vi "draw_position_overlay.vi"(7 "pixel look-up mode":T1, 8 "error in (no error)":errorcluster, 9 "pixel positions":T2[](array[typedef]), 10 "frame index":i32, 11 "ImageCollection in":refnum<class "ImageCollection.lvclass">) -> (0 "error out":errorcluster, 2 "Image.lvclass":refnum<class "Image.lvclass">, 3 "ImageCollection out":refnum<class "ImageCollection.lvclass">)   [LabVIEW 2010, in "ImageCollection.lvclass"]
uses:
  ImageCollection.lvclass
  Image/Image/Image.lvclass
  pixel_position_cluster.ctl
  enumerations/pixel_lookup_mode_enum.ctl
  Image/Image/pixel_position_cluster.ctl
  Image/Image/pixel_positions_cluster.ctl
  ImageCollection.lvclass/ImageCollection.ctl
panel:
  out "is line on current plane?":bool
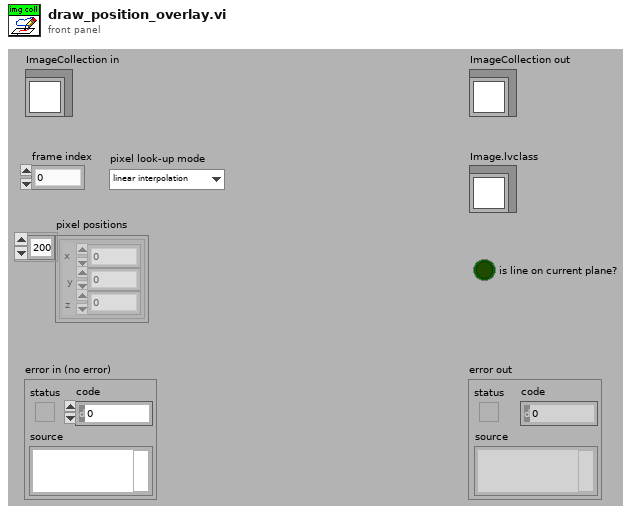
[diagram p1: front panel]
types:
  T1 = typedef "pixel_lookup_mode_enum.ctl" = enum16{"linear interpolation", "binary search"}
  T2 = typedef "ImageCollection.lvclass/pixel_position_cluster.ctl" = cluster{"x":dbl, "y":dbl, "z ":dbl}
  T3 = typedef "Image.lvclass/pixel_position_cluster.ctl" = cluster{"x":dbl, "y":dbl}
  T4 = typedef "Image.lvclass/pixel_positions_cluster.ctl" = cluster{"x":dbl[], "y":dbl[], "z":dbl}
  T5 = typedef "ImageCollection.lvclass/pixel_positions_cluster.ctl" = cluster{"x":dbl[], "y":dbl[], "z":dbl[]}
  T6 = cluster{"Line End Points":cluster{"X":dbl, "Y":dbl}[]}
  T7 = cluster{"Line End Points":cluster{"X":dbl, "Y":dbl}[]}[]
  T8 = typedef "IMAQ Image.ctl" = refnum<image>
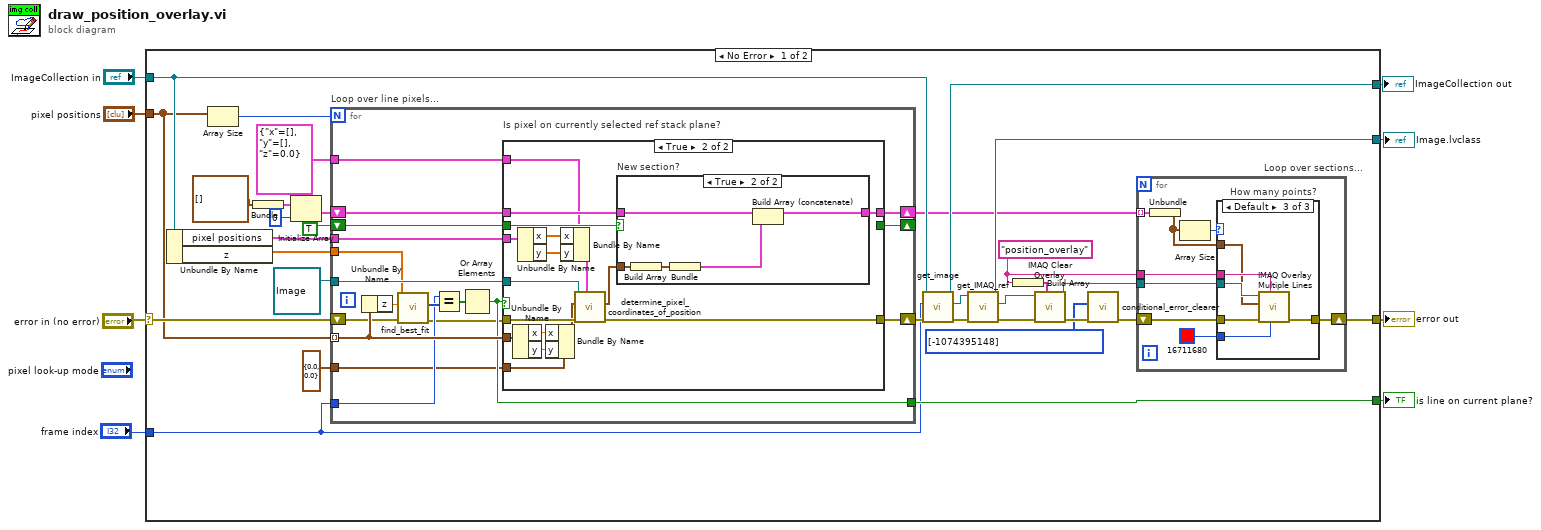
[diagram p0: block diagram]
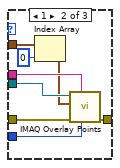
[diagram p3: hidden frame]
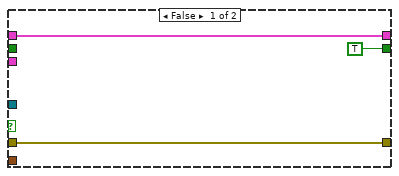
[diagram p4: hidden frame]
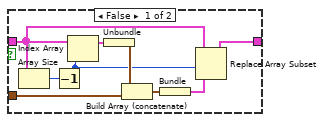
[diagram p5: hidden frame]
diagram:
  n1 = case shown="No Error" "error in (no error)" {
    selector: "error in (no error)" -> [w35 w116]
    tunnel: "frame index" -> [w12 _]
    tunnel: [w39 w116] -> w6
    tunnel: [w38 _] -> w8
    tunnel: "pixel positions" -> [w19 _]
    tunnel: "ImageCollection in" -> [w33 w115]
    tunnel: [w32 w115] -> w4
    tunnel: [w26 _] -> w2
    frame No Error {
      w23 = "position_overlay"
      n2 = Unbundle By Name(w33) -> ("pixel positions"=w37:T5, "z"=w27:dbl[])
      n3 = Array Size(array=w19) -> (size(s)=w36:i32)
      n4 = Bundle("Line End Points"=cluster{"X":dbl, "Y":dbl}[] []) -> (w10:T6)  [unwired: 1 in]
      n5 = Initialize Array(w10, 0 ("dimension size")) -> (w9:T7)
      n6 = for "Loop over line pixels..." {
        N: w36 -> [_]
        shift-right: [w80] -> w34
        shift-left: w35 -> [w71]
        shift-right: [w78] -> w20
        shift-left: w9 -> [w79]
        tunnel: w37 -> [w77]
        tunnel: w12 -> [w67]
        tunnel: w27 -> [w70]
        tunnel: [w66] -> w38
        tunnel: w19 -> [w76] mode=indexing
        shift-right: [w74] -> _
        shift-left: TRUE -> [w75]
        tunnel: T4 {"x"=[], "y"=[], "z"=0.0} ("pixel positions") -> [w73]
        tunnel: refnum<class "Image.lvclass"> refnum ("Image.lvclass") -> [w72]
        tunnel: T3 {"x"=0.0, "y"=0.0} ("pixel position") -> [w63]
        n7 = Unbundle By Name(w76) -> ("z"=w69:dbl)
        n8 = call "find_best_fit.vi"("error in (no error)"=w71, "value to be found"=w69, "search space"=w70) -> ("error out"=w64:errorcluster, "indices of fits"=w68:i32[])  [unwired: 6 in, 1 out]
        n9 = Equal?(x=w67, y=w68) -> (x = y?=w65:bool[])
        n10 = Or Array Elements(Boolean array=w65) -> (logical OR=w66:bool)
        n11 = case "Is pixel on currently selected ref stack plane?" shown="True" w66 {
          tunnel: w64 -> [w83 w100]
          tunnel: [w83 w99] -> w80
          tunnel: w79 -> [w82 w97]
          tunnel: [w82 w98] -> w78
          tunnel: w77 -> [_ w92]
          tunnel: w76 -> [_ w88]
          tunnel: w75 -> [_ w95]
          tunnel: [TRUE _] -> w74
          tunnel: w73 -> [_ w94]
          tunnel: w72 -> [_ w93]
          tunnel: w63 -> [_ w87]
          frame False {
          }
          frame True {
            n12 = Unbundle By Name(w88) -> ("x"=w86:dbl, "y"=w85:dbl)
            n13 = Unbundle By Name(w92) -> ("x"=w91:dbl[], "y"=w90:dbl[])
            n14 = Bundle By Name(cluster=w87, "x"=w86, "y"=w85) -> (w84:T3)
            n15 = Bundle By Name(cluster=w94, "x"=w91, "y"=w90) -> (w89:T4)
            n16 = call "determine_pixel_coordinates_of_position.vi"("pixel positions"=w89, "error in (no error)"=w100, "pixel position"=w84, "Image in"=w93) -> ("error out"=w99:errorcluster, "Point Coordinates"=w96:cluster{"X":dbl, "Y":dbl})  [unwired: 5 in, 1 out]
            n17 = case "New section?" shown="True" w95 {
              tunnel: [w101 w114] -> w98
              tunnel: w97 -> [w104 w113]
              tunnel: w96 -> [w107 w112]
              frame False {
                n18 = Array Size(array=w104) -> (size(s)=w109:i32)
                n19 = Decrement(x=w109) -> (x-1=w102:i32)
                n20 = Index Array(array=w104, index=w102) -> (element=w108:T6)
                n21 = Unbundle(w108) -> ("Line End Points"=w106:cluster{"X":dbl, "Y":dbl}[])
                n22 = Build Array (concatenate)(w106, w107) -> (w105:cluster{"X":dbl, "Y":dbl}[])
                n23 = Bundle(w105) -> (w103:cluster{cluster{"X":dbl, "Y":dbl}[]})  [unwired: 1 in]
                n24 = Replace Array Subset(array=w104, new element=w103, index=w102) -> (w101:T7)
              }
              frame True {
                n25 = Build Array(w112) -> (w111:cluster{"X":dbl, "Y":dbl}[])
                n26 = Bundle(w111) -> (w110:cluster{cluster{"X":dbl, "Y":dbl}[]})  [unwired: 1 in]
                n27 = Build Array (concatenate)(w113, w110) -> (w114:T7)
              }
            }
          }
        }
      }
      n28 = call-dynamic "get_image.vi"("error in (no error)"=w34, "index"=w12, "ImageCollection in"=w33) -> ("error out"=w31:errorcluster, "Image.lvclass"=w29:refnum<class "Image.lvclass">, "ImageCollection out"=w32:refnum<class "ImageCollection.lvclass">)  [unwired: 6 in]
      n29 = call-dynamic "get_IMAQ_ref.vi"("error in (no error)"=w31, "Image.lvclass in"=w29) -> ("error out"=w30:errorcluster, "Image"=w28:T8, "Image.lvclass out"=w26:refnum<class "Image.lvclass">)  [unwired: 5 in, 2 out]
      n30 = Build Array(w23) -> (w21:string[])
      n31 = call "IMAQ Clear Overlay"("Groups"=w21, "error in (no error)"=w30, "Image"=w28) -> ("error out"=w15:errorcluster, "Image Out"=w22:T8)  [unwired: 7 in]
      n32 = call "conditional_error_clearer.vi"("error in (no error)"=w15, "array of clearable error codes"=i32[] [-1074395148]) -> ("error out"=w14:errorcluster)  [unwired: 9 in]
      n33 = for "Loop over sections..." {
        tunnel: w22 -> [w46]
        shift-right: [w40] -> w39
        shift-left: w14 -> [w47]
        tunnel: w23 -> [w45]
        tunnel: w20 -> [w44] mode=indexing
        n34 = Unbundle(w44) -> ("Line End Points"=w43:cluster{"X":dbl, "Y":dbl}[])
        n35 = Array Size(array=w43) -> (size(s)=w42:i32)
        n36 = case "How many points?" shown="Default" w42 {
          tunnel: w47 -> [w48 w56 w61]
          tunnel: w46 -> [_ w54 w60]
          tunnel: w45 -> [_ w53 w59]
          tunnel: w43 -> [_ w51 w58]
          tunnel: u32 16711680 ("Color") -> [_ w52 w57]
          tunnel: [w48 w55 w62] -> w40
          frame 0 {
          }
          frame 1 {
            n37 = Index Array(array=w51, index=0) -> (element=w49:cluster{"X":dbl, "Y":dbl})
            n38 = call "IMAQ Overlay Points"("Color"=w52, "Group"=w53, "error in (no error)"=w56, "Point"=w49, "Image"=w54) -> ("error out"=w55:errorcluster)  [unwired: 5 in, 1 out]
          }
          frame Default {
            n39 = call "IMAQ Overlay Multiple Lines"("Color"=w57, "Group"=w59, "error in (no error)"=w61, "Line End Points"=w58, "Image"=w60) -> ("error out"=w62:errorcluster)  [unwired: 5 in, 1 out]
          }
        }
      }
    }
    frame Error {
    }
  }
  "error out" <- w6
  "ImageCollection out" <- w4
  "Image.lvclass" <- w2
  "is line on current plane?" <- w8
